vi "Resize.Resize 3 Charts within Tab Ctrl.vi"(4 "Plot Cnt":i32=4, 5 "Pix from Bottom":i32, 6 "Min Size":cluster{"Width":i32, "Height":i32}={"Width"=300, "Height"=50}, 7 "Pix from Right":i32, 8 "error in":errorcluster, 9 "Aspect Ratio":cluster{"W/H":dbl, "Enable":bool}={"W/H"=1.0, "Enable"=FALSE} {"W/H" format="%.2g"}, 10 "Charts In":refnum<vi>[](array[refnum]), 11 "Tab Ctrl":refnum<vi>) -> (0 "error out":errorcluster, 2 "Charts Out":refnum<vi>[](array[refnum]), 3 "Tab Ctrl Out":refnum<vi>)   [LabVIEW 2024, in "EQMF.lvlib" / "Controls.lvlib"]
uses:
  Controls.lvlib
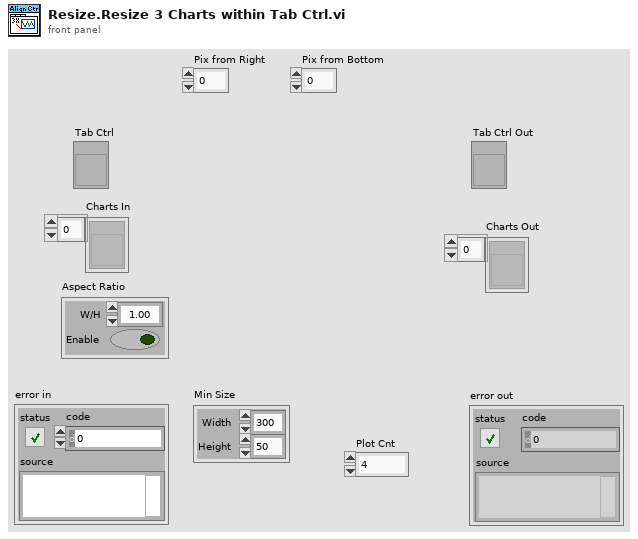
[diagram p1: front panel]
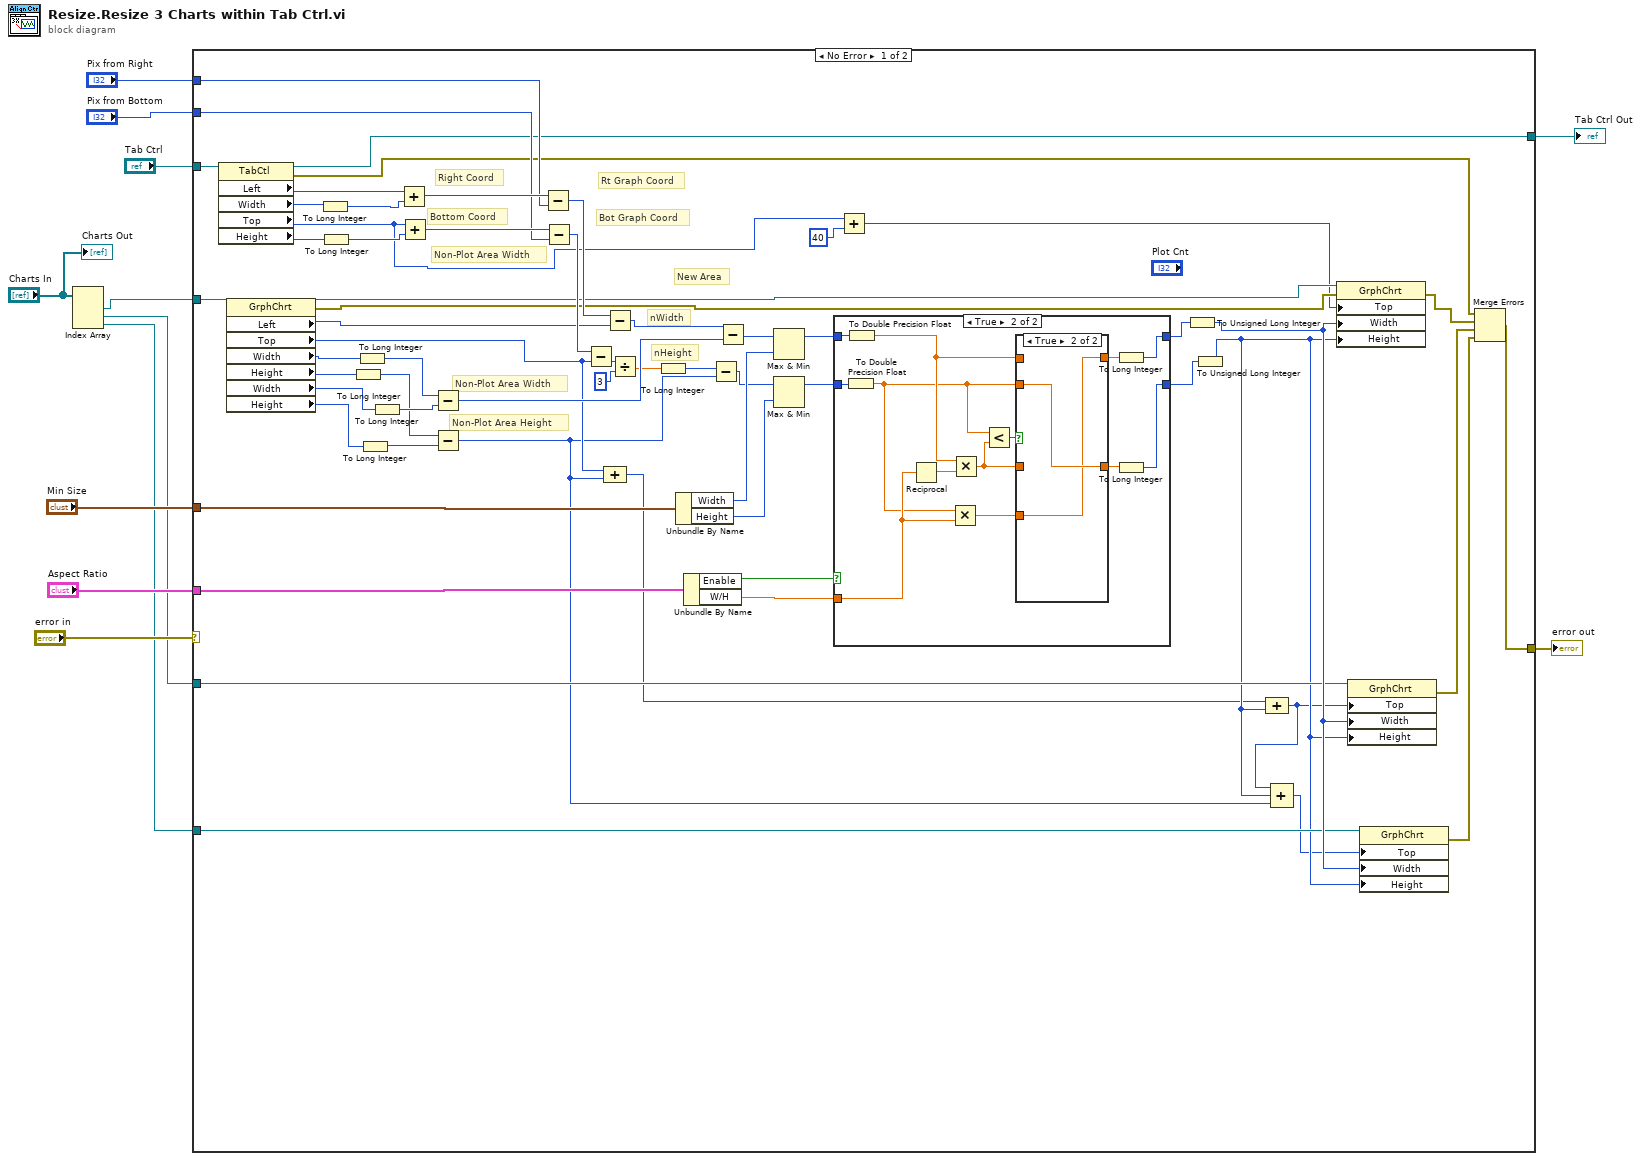
[diagram p0: block diagram]
diagram:
  n1 = Index Array(array="Charts In") -> (element #1=w4:refnum<vi>, element #2=w2:refnum<vi>, element #3=w1:refnum<vi>)  [unwired: 3 in]
  n2 = case shown="No Error" "error in" {
    selector: "error in" -> [_ w92]
    tunnel: "Pix from Right" -> [w57 _]
    tunnel: "Pix from Bottom" -> [w56 _]
    tunnel: [w48 w92] -> w10
    tunnel: "Min Size" -> [w47 _]
    tunnel: "Aspect Ratio" -> [w42 _]
    tunnel: "Tab Ctrl" -> [w39 w93]
    tunnel: w4 -> [w38 _]
    tunnel: [w35 w93] -> w6
    tunnel: w2 -> [w25 _]
    tunnel: w1 -> [w24 _]
    frame No Error {
      # "nHeight"
      # "nWidth"
      # "New Area"
      # "Bot Graph Coord"
      # "Rt Graph Coord"
      # "Non-Plot Area Width"
      # "Bottom Coord"
      # "Right Coord"
      # "Non-Plot Area Height"
      # "Non-Plot Area Width"
      n3 = property on="Property Node" class="TabCtl"(reference=w39) -> (reference out=w35:refnum<vi>, error out=w37:errorcluster, "Left"=w61:i32, "Width"=w63:u32, "Top"=w15:i32, "Height"=w62:u32)  [unwired: 1 in]
      n4 = property on="Property Node" class="GrphChrt"(reference=w38) -> (reference out=w50:refnum<vi>, error out=w49:errorcluster, "Left"=w53:i32, "Top"=w22:i32, "Width"=w60:u32, "Height"=w72:u32, "Width"=w71:u32, "Height"=w70:u32)  [unwired: 1 in]
      n5 = To Long Integer(number=w63) -> (32bit integer=w64:i32)
      n6 = To Long Integer(number=w62) -> (32bit integer=w65:i32)
      n7 = To Long Integer(number=w72) -> (32bit integer=w67:i32)
      n8 = To Long Integer(number=w60) -> (32bit integer=w68:i32)
      n9 = To Long Integer(number=w70) -> (32bit integer=w66:i32)
      n10 = To Long Integer(number=w71) -> (32bit integer=w69:i32)
      n11 = Add(x=w61, y=w64) -> (x+y=w58:i32)
      n12 = Add(x=w15, y=w65) -> (x+y=w59:i32)
      n13 = Subtract(x=w68, y=w69) -> (x-y=w51:i32)
      n14 = Subtract(x=w67, y=w66) -> (x-y=w20:i32)
      n15 = Subtract(x=w58, y=w57) -> (x-y=w55:i32)
      n16 = Subtract(x=w59, y=w56) -> (x-y=w54:i32)
      n17 = Subtract(x=w54, y=w22) -> (x-y=w32:i32)
      n18 = Compound Arithmetic op=ADD(w22, w20) -> (w21:i32)
      n19 = Subtract(x=w55, y=w53) -> (x-y=w52:i32)
      n20 = Divide(x=w32, y=3) -> (x/y=w30:dbl)
      n21 = To Long Integer(number=w30) -> (32bit integer=w29:i32)
      n22 = Unbundle By Name(w47) -> ("Width"=w46:i32, "Height"=w45:i32)
      n23 = Unbundle By Name(w42) -> ("Enable"=w41:bool, "W/H"=w40:dbl)
      n24 = Subtract(x=w29, y=w20) -> (x-y=w44:i32)
      n25 = Subtract(x=w52, y=w51) -> (x-y=w43:i32)
      n26 = Max & Min(x=w43, y=w46) -> (max(x,y)=w28:i32)  [unwired: 1 out]
      n27 = Max & Min(x=w44, y=w45) -> (max(x,y)=w27:i32)  [unwired: 1 out]
      n28 = case shown="True" w41 {
        tunnel: w28 -> [w74 w87]
        tunnel: w27 -> [w73 w86]
        tunnel: [w74 w78] -> w34
        tunnel: [w73 w79] -> w33
        tunnel: w40 -> [_ w84]
        frame False {
        }
        frame True {
          n29 = To Double Precision Float(number=w86) -> (double precision float=w76:dbl)
          n30 = To Double Precision Float(number=w87) -> (double precision float=w83:dbl)
          n31 = Reciprocal(x=w84) -> (1/x=w85:dbl)
          n32 = Multiply(x=w76, y=w84) -> (x*y=w75:dbl)
          n33 = Multiply(x=w83, y=w85) -> (x*y=w82:dbl)
          n34 = Less?(x=w76, y=w82) -> (x < y?=w81:bool)
          n35 = case shown="True" w81 {
            tunnel: w83 -> [w89 _]
            tunnel: w82 -> [w88 _]
            tunnel: [w89 w90] -> w77
            tunnel: [w88 w91] -> w80
            tunnel: w76 -> [_ w91]
            tunnel: w75 -> [_ w90]
            frame False {
            }
            frame True {
            }
          }
          n36 = To Long Integer(number=w77) -> (32bit integer=w78:i32)
          n37 = To Long Integer(number=w80) -> (32bit integer=w79:i32)
        }
      }
      n38 = Add(x=w15, y=40) -> (x+y=w13:i32)
      n39 = To Unsigned Long Integer(number=w34) -> (unsigned 32bit integer=w26:u32)
      n40 = To Unsigned Long Integer(number=w33) -> (unsigned 32bit integer=w23:u32)
      n41 = Compound Arithmetic op=ADD(w21, w23) -> (w19:u32)
      n42 = Compound Arithmetic op=ADD(w19, w23, w20) -> (w18:u32)
      n43 = property on="Property Node" class="GrphChrt"(reference=w50, error in=w49, "Top"=w13, "Width"=w26, "Height"=w23) -> (error out=w36:errorcluster)  [unwired: 1 out]
      n44 = property on="Property Node" class="GrphChrt"(reference=w25, "Top"=w19, "Width"=w26, "Height"=w23) -> (error out=w17:errorcluster)  [unwired: 1 in, 1 out]
      n45 = property on="Property Node" class="GrphChrt"(reference=w24, "Top"=w18, "Width"=w26, "Height"=w23) -> (error out=w16:errorcluster)  [unwired: 1 in, 1 out]
      n46 = Merge Errors(w37, w36, w17, w16) -> (w48:errorcluster)
    }
    frame Error {
    }
  }
  "error out" <- w10
  "Tab Ctrl Out" <- w6
  "Charts Out" <- "Charts In"
